vi "MagRetBypass_Main.vi"() -> ()   [LabVIEW 2019]
uses:
  MagRetBypass_Global.vi
panel:
  in  "full_close":bool
  in  "full_open":bool
  out "opening":dbl(slide) caption="Opening (%)" scale=0.0..100.0
  in  "set_opening":bool
  in  "set_point":dbl caption="Set point" min=0.0 max=100.0 step=0.01 format="%.2f"
  out "Chart":waveform(dbl)[](graph)
  out "status_log":bool caption="Status"
  out "status":bool caption="Status"
  in  "Logging":bool=TRUE
  in  "stop":bool
  out "Last Measurement":timestamp format="%<%Y-%m-%d %H:%M:%S>T"
  in  "VISA":refnum<visa-resource-name>="COM39"
  in  "Readout Interval":i32=1
  # "Magnet Return Bypass"
  # "sec"
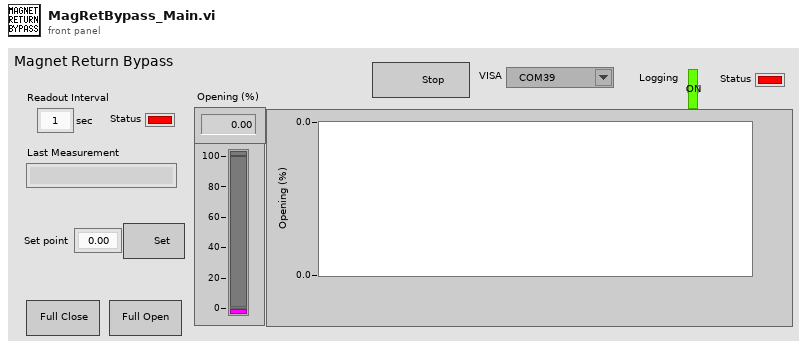
[diagram p1: front panel]
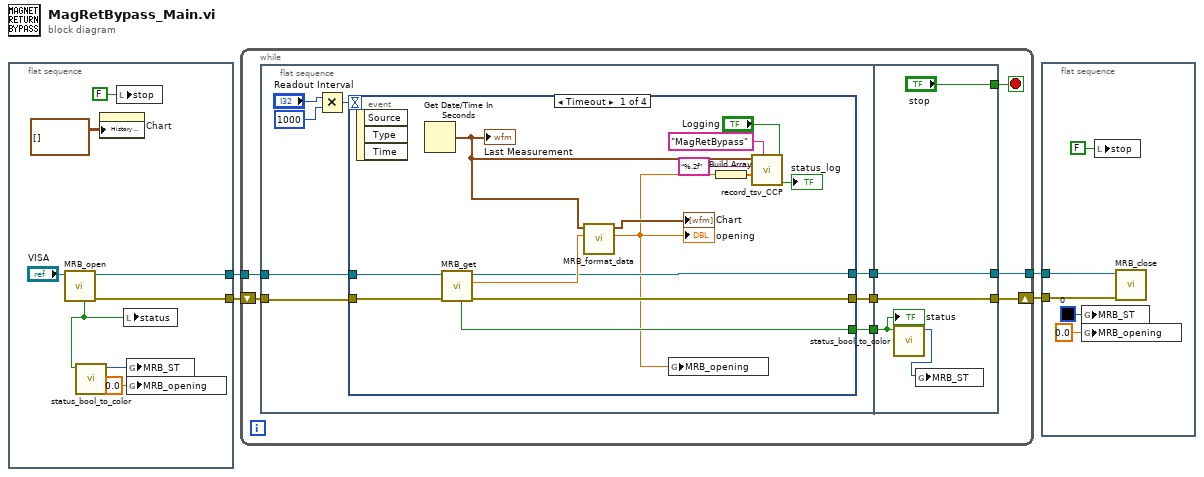
[diagram p0: block diagram]
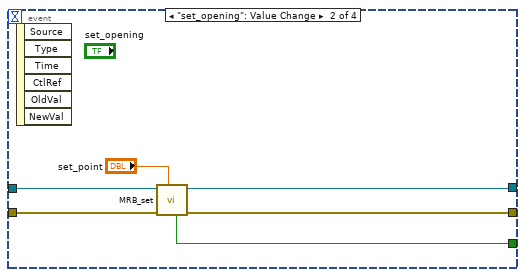
[diagram p2: hidden frame]
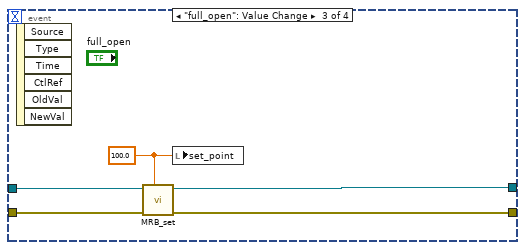
[diagram p3: hidden frame]
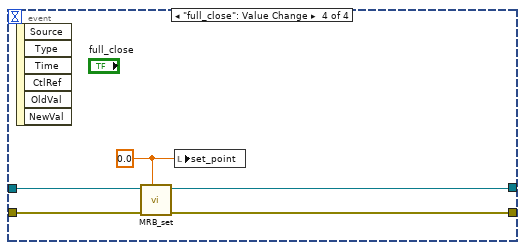
[diagram p4: hidden frame]
diagram:
  n1 = flat-sequence {
    tunnel: [w8] -> w4
    tunnel: [w7] -> w3
    frame #0 {
      n2 = call "MRB_open.vi"("thcd_visa"="VISA") -> ("err_out"=w7:errorcluster, "thcd_visa"=w8:refnum<visa-resource-name>, "status"=w5:bool)  [unwired: 8 in]
      n3 = call "status_bool_to_color.vi"("status_bool_1"=w5) -> ("status_color"=w6:u32)  [unwired: 10 in]
      n4 = property on="Chart" class="WFChart (strict)"("History Data"=waveform(dbl)[][] []) -> ()  [unwired: 2 in, 2 out]
      n5 = local write "stop"(FALSE ("stop")) -> ()
      n6 = local write "status"(w5) -> ()
      n7 = global write "MagRetBypass_Global.vi" "MRB_ST"(w6) -> ()
      n8 = global write "MagRetBypass_Global.vi" "MRB_opening"(0.0 ("TPG361_p")) -> ()
    }
  }
  n9 = while {
    tunnel: w4 -> [w20]
    tunnel: [w19] -> w2
    shift-right: [w15] -> w1
    shift-left: w3 -> [w18]
    stop <- w16 stop-if-true
    n10 = flat-sequence {
      tunnel: w20 -> [w28]
      tunnel: w18 -> [w26]
      tunnel: [w27] -> w17
      tunnel: [w25] -> w14
      tunnel: [w24] -> w13
      tunnel: [w63] -> w19
      tunnel: w17 -> [w63]
      tunnel: ["stop"] -> w16
      tunnel: [w62] -> w15
      tunnel: w14 -> [w62]
      tunnel: w13 -> [w59]
      frame #0 {
        n11 = Multiply(x="Readout Interval", y=1000) -> (x*y=w23:i32)
        n12 = event shown="[0] Timeout" {
          selector: _ -> [_ _ _ _]
          dyn-events: _ -> [_ _ _ _]
          timeout: w23 -> [_ _ _ _]
          tunnel: w28 -> [w36 w46 w53 w58]
          tunnel: [w31 w45 w52 w57] -> w27
          tunnel: w26 -> [w39 w48 w51 w56]
          tunnel: [w34 w47 w50 w55] -> w25
          tunnel: [w30 w43 _ _] -> w24
          event Timeout {
            n13 = event-data() -> ()  [unwired: 1 in, 3 out]
            n14 = Get Date/Time In Seconds() -> (seconds since 1Jan1904=w37:timestamp)
            "Last Measurement" <- w37
            n15 = call "MRB_get.vi"("err_in"=w39, "visa_in"=w36) -> ("err_out"=w34:errorcluster, "opening"=w35:dbl, "visa_out"=w31:refnum<visa-resource-name>, "status"=w30:bool)  [unwired: 6 in]
            n16 = call "MRB_format_data.vi"("pressure"=w35, "time"=w37) -> ("pressure_out"=w29:dbl, "waveform_array"=→"Chart":waveform(dbl)[])  [unwired: 8 in]
            "opening" <- w29
            n17 = global write "MagRetBypass_Global.vi" "MRB_opening"(w29) -> ()
            n18 = Build Array(w29) -> (w33:dbl[])
            n19 = call "record_tsv_CCP.vi"("logging_on"="Logging", "folder_name"="MagRetBypass", "value_array"=w33, "format"="%.2f", "time"=w37) -> ("status"=→"status_log":bool)  [unwired: 5 in, 1 out]
          }
          event "set_opening": Value Change {
            n20 = event-data() -> ()  [unwired: 1 in, 6 out]
            n21 = call "MRB_set.vi"("set_point"="set_point", "err_in"=w48, "visa_in"=w46) -> ("err_out"=w47:errorcluster, "visa_out"=w45:refnum<visa-resource-name>, "status"=w43:bool)  [unwired: 5 in, 1 out]
          }
          event "full_open": Value Change {
            w49 = 100.0 ("set_point")
            n22 = event-data() -> ()  [unwired: 1 in, 6 out]
            n23 = call "MRB_set.vi"("set_point"=w49, "err_in"=w51, "visa_in"=w53) -> ("err_out"=w50:errorcluster, "visa_out"=w52:refnum<visa-resource-name>)  [unwired: 5 in, 2 out]
            n24 = local write "set_point"(w49) -> ()
          }
          event "full_close": Value Change {
            w54 = 0.0 ("set_point")
            n25 = event-data() -> ()  [unwired: 1 in, 6 out]
            n26 = call "MRB_set.vi"("set_point"=w54, "err_in"=w56, "visa_in"=w58) -> ("err_out"=w55:errorcluster, "visa_out"=w57:refnum<visa-resource-name>)  [unwired: 5 in, 2 out]
            n27 = local write "set_point"(w54) -> ()
          }
        }
      }
      frame #1 {
        n28 = call "status_bool_to_color.vi"("status_bool_1"=w59) -> ("status_color"=w60:u32)  [unwired: 10 in]
        n29 = global write "MagRetBypass_Global.vi" "MRB_ST"(w60) -> ()
        "status" <- w59
      }
    }
  }
  n30 = flat-sequence {
    tunnel: w2 -> [w68]
    tunnel: w1 -> [w67]
    frame #0 {
      n31 = global write "MagRetBypass_Global.vi" "MRB_ST"(u32 0 ("TPG361_ST")) -> ()
      n32 = global write "MagRetBypass_Global.vi" "MRB_opening"(0.0 ("TPG361_p")) -> ()
      n33 = local write "stop"(FALSE ("stop")) -> ()
      n34 = call "MRB_close.vi"("error in (no error)"=w67, "VISA session"=w68) -> ()  [unwired: 9 in, 1 out]
    }
  }
